vi "DMCConfiguatorGui.CreateDMC.vi"(9 "Plate":T1, 10 "Variant":T2={"State"=enum."Init", "ImgPath"=path "", "WabcoPlate"="", "WabcoProduct"="", "ClientProduct"="", "ClientPlate"="", "TotalQuantity"=0, "Serial"=0, "Wabco"={"LaserJob"="", "AdditionalTxt"="037", "FactoryCode"="", "RevID"=0, "ForkID"=0, "FailuresLimit"=0, "GlobalCnt"=0, "CheckDM"=FALSE, "SerialFormat"=enum."000001 - 499999", "CoordA"={"X"=0.0, "Y"=0.0, "Angle"=0.0}, "CoordB"={"X"=0.0, "Y"=0.0, "Angle"=0.0}, "DMCconfig"=0}, "Client"={"LaserJob"="", "AdditionalTxt"="", "FactoryCode"="037", "RevID"=0, "ForkID"=0, "FailuresLimit"=0, "GlobalCnt"=0, "CheckDM"=FALSE, "SerialFormat"=enum."000001 - 499999", "CoordA"={"X"=0.0, "Y"=0.0, "Angle"=0.0}, "CoordB"={"X"=0.0, "Y"=0.0, "Angle"=0.0}, "DMCconfig"=0}}, 11 "DMCConfig":T7) -> (1 "found":bool, 3 "DMC":string)   [LabVIEW 2015]
uses:
  DMCConfiguatorGui.ConfigData.ctl
  DMCConfiguatorGui.Component.ctl
  DMCConfiguatorGui.Type.ctl
  DMCConfiguatorGui.Var.ctl
  Logger/Logger.Variant.Sets.ctl
  Station/Station.Changeover.State.vi
  Station/Station.Plate.Properties.ctl
  Sequence/Sequence.Code.SerialFormat.ctl
  Drivers/V7310/LowLevel/V7310.Job.Sets.ctl
  Sequence/Sequence.PlateType.ctl
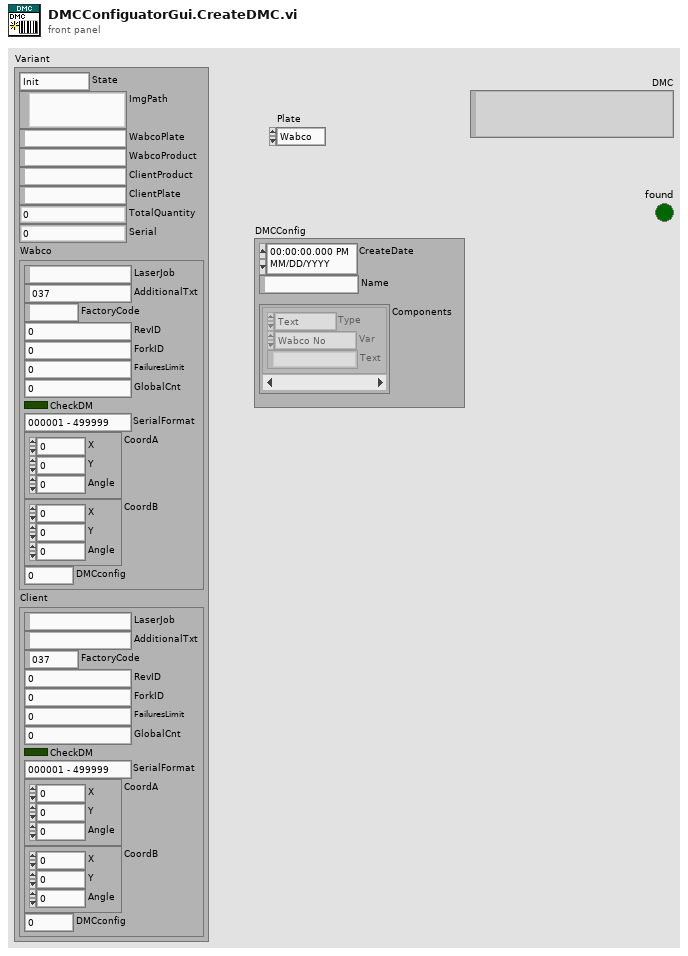
[diagram p1: front panel]
types:
  T1 = typedef "Sequence.PlateType.ctl" = enum16{"Wabco", "Client"}
  T2 = typedef "Logger.Variant.Sets.ctl" = cluster{"State":T3, "ImgPath":path, "WabcoPlate":string, "WabcoProduct":string, "ClientProduct":string, "ClientPlate":string, "TotalQuantity":u16, "Serial":i32, "Wabco":T4, "Client":T4}
  T3 = typedef "Station.Changeover.State.vi" = enum16{"Init", "Scaning", "NOK", "Wait for ack", "Ready"}
  T4 = typedef "Station.Plate.Properties.ctl" = cluster{"LaserJob":string, "AdditionalTxt":string, "FactoryCode":string, "RevID":u8, "ForkID":u8, "FailuresLimit":u16, "GlobalCnt":i32, "CheckDM":bool, "SerialFormat":T5, "CoordA":T6, "CoordB":T6, "DMCconfig":i32}
  T5 = typedef "Sequence.Code.SerialFormat.ctl" = enum8{"", "000001 - 499999", "500001 - 999999", "0000001 - 4999999", "5000001 - 9999999"}
  T6 = typedef "V7310.Job.Sets.ctl" = cluster{"X":dbl, "Y":dbl, "Angle":dbl}
  T7 = typedef "DMCConfiguatorGui.ConfigData.ctl" = cluster{"CreateDate":timestamp, "Name":string, "Components":T8[]}
  T8 = typedef "DMCConfiguatorGui.Component.ctl" = cluster{"Type":T9, "Var":T10, "Text":string}
  T9 = typedef "DMCConfiguatorGui.Type.ctl" = enum8{"Text", "Variable"}
  T10 = typedef "DMCConfiguatorGui.Var.ctl" = enum8{"-", "Wabco No", "Client No", "Serial", "Date"}
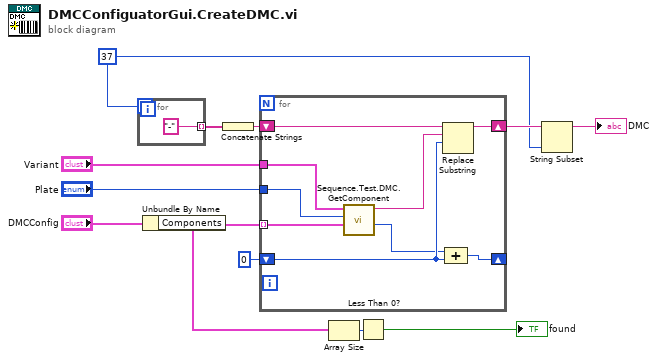
[diagram p0: block diagram]
diagram:
  w6 = 37 ("Size (37)")
  n1 = for {
    N: w6 -> [_]
    tunnel: ["-"] -> w12 mode=indexing
  }
  n2 = Unbundle By Name("DMCConfig") -> ("Components"=w9:T8[])
  n3 = Concatenate Strings(w12) -> (w11:string)
  n4 = for {
    tunnel: w9 -> [w18] mode=indexing
    shift-right: [w21] -> w10
    shift-left: w11 -> [w22]
    tunnel: "Variant" -> [w16]
    shift-right: [w19] -> _
    shift-left: u8 0 -> [w20]
    tunnel: "Plate" -> [w15]
    n5 = call "Sequence.Test.DMC.GetComponent.vi"("Component"=w18, "Plate"=w15, "OrderSets"=w16) -> ("max size"=w17:i32, "Value"=w14:string)  [unwired: 6 in, 1 out]
    n6 = Replace Substring(3:w20, 4:w14, 5:w22) -> (1:w21:string)  [unwired: 1 in, 1 out]
    n7 = Compound Arithmetic op=ADD(w17, w20) -> (w19:i32)
  }
  n8 = Array Size(array=w9) -> (size(s)=w8:i32)
  n9 = Less Than 0?(x=w8) -> (x < 0?=→"found":bool)
  n10 = String Subset(string=w10, length (rest)=w6) -> (substring=→"DMC":string)  [unwired: 1 in]
